vi "Transmit Command NoErr.vi"(8 "error in":errorcluster, 10 "Command":string, 11 "3300 in":refnum<class "3300.lvclass">) -> (0 "error out":errorcluster, 3 "3300 out":refnum<class "3300.lvclass">)   [LabVIEW 2019, in "3300.lvlib" / "3300.lvclass"]
doc: "This routine sends a command to the 3300, but does not query error status. \nThis is intended for measurement query commands where sending the query should immediately be followed by a read of the queried data, error checks will interrupt the query action result in a guaranteed error."
uses:
  Library/3300.lvclass
  Library/3300.lvclass/3300.ctl
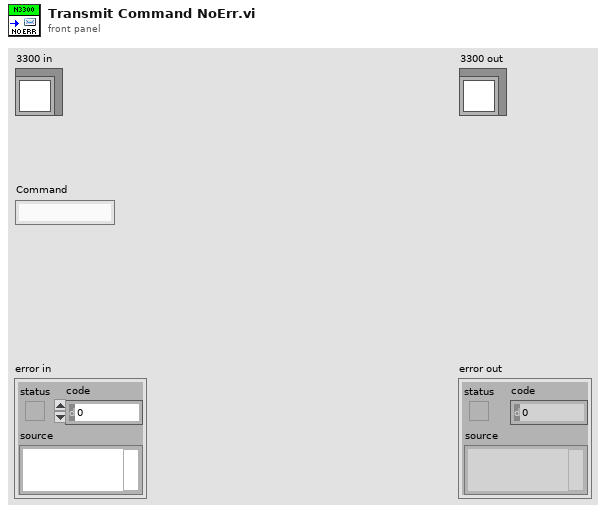
[diagram p1: front panel]
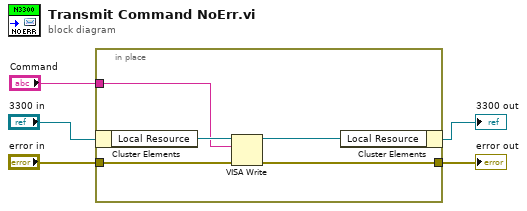
[diagram p0: block diagram]
diagram:
  n1 = in-place {
    in-place-border: "Command" -> [w9]
    in-place-border: "error in" -> [w8]
    in-place-border: [w6] -> w3
    n2 = in-place-cluster #1("3300 in") -> ("Local Resource"=w10:refnum<visa-resource-name>)
    n3 = VISA Write(VISA resource name=w10, write buffer=w9, error in (no error)=w8) -> (VISA resource name out=w7:refnum<visa-resource-name>, error out=w6:errorcluster)  [unwired: 1 out]
    n4 = in-place-cluster #1("Local Resource"=w7) -> (→"3300 out":refnum<class "3300.lvclass">)
  }
  "error out" <- w3
